vi "9-while loop stop.vi"() -> ()   [LabVIEW 2018]
panel:
  in  "OK Button":bool
  out "Numeric":i32
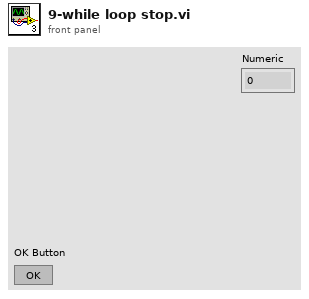
[diagram p1: front panel]
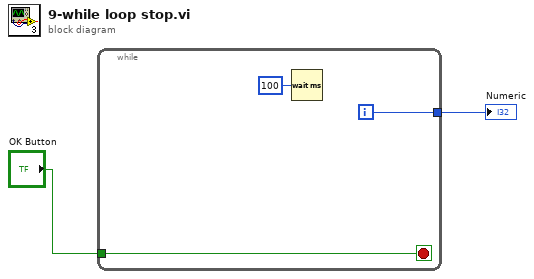
[diagram p0: block diagram]
diagram:
  n1 = while {
    tunnel: [w4] -> w2
    tunnel: "OK Button" -> [w3]
    i -> [w4]
    stop <- w3 stop-if-true
    n2 = Wait (ms)(milliseconds to wait=u32 100) -> ()  [unwired: 1 out]
  }
  "Numeric" <- w2
